vi "Set AO Gain Property Node Global.vi"(9 "AO Gain (Property Node)":dbl[](array[numeric])=[0.0, 0.0, 0.0, -4.440892098500626e-16, 0.0, 0.0, 0.0, 0.0, 0.0, 0.0] min=-40.0 max=0.0 step=20.0) -> ()   [LabVIEW 2015]
uses:
  PXI Globals.vi
panel:
  # "PXI DAQ MUST BE STOPPED AND RESTARTED FOR GAIN TO CHANGE."
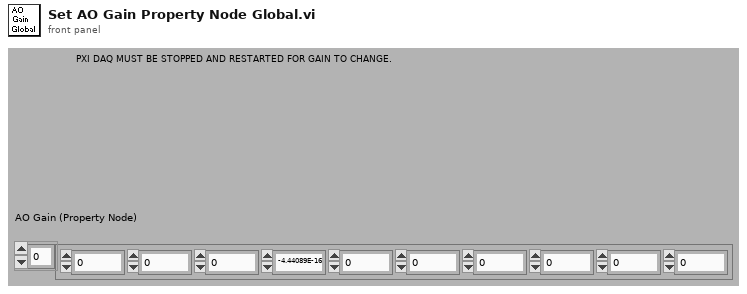
[diagram p1: front panel]
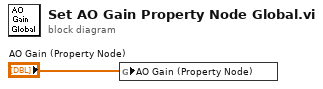
[diagram p0: block diagram]
diagram:
  n1 = global write "PXI Globals.vi" "AO Gain (Property Node)"("AO Gain (Property Node)") -> ()
